vi "are there nodes with unexplored children.vi"(8 "error in (no error)":errorcluster, 11 "current_path":T1[](array[typedef])) -> (0 "error out":errorcluster, 3 "T = there is at least one node with at least one unexplored child":bool)   [LabVIEW 2021, in "Project Euler.lvlib"]
uses:
  Project Euler.lvlib
  lattice_path_node.ctl
  lattice_path_direction.ctl
panel:
  out "node number":i32
  # "Development\ncontrols/indicators useful for development and testing, but which are not outputs of the VI"
  # "Input\nInputs to the VI"
  # "Output\nOutputs of the VI"
  # "Description\n\nBlank VI with error handling case. \n\nSummarize the use of this VI in this space."
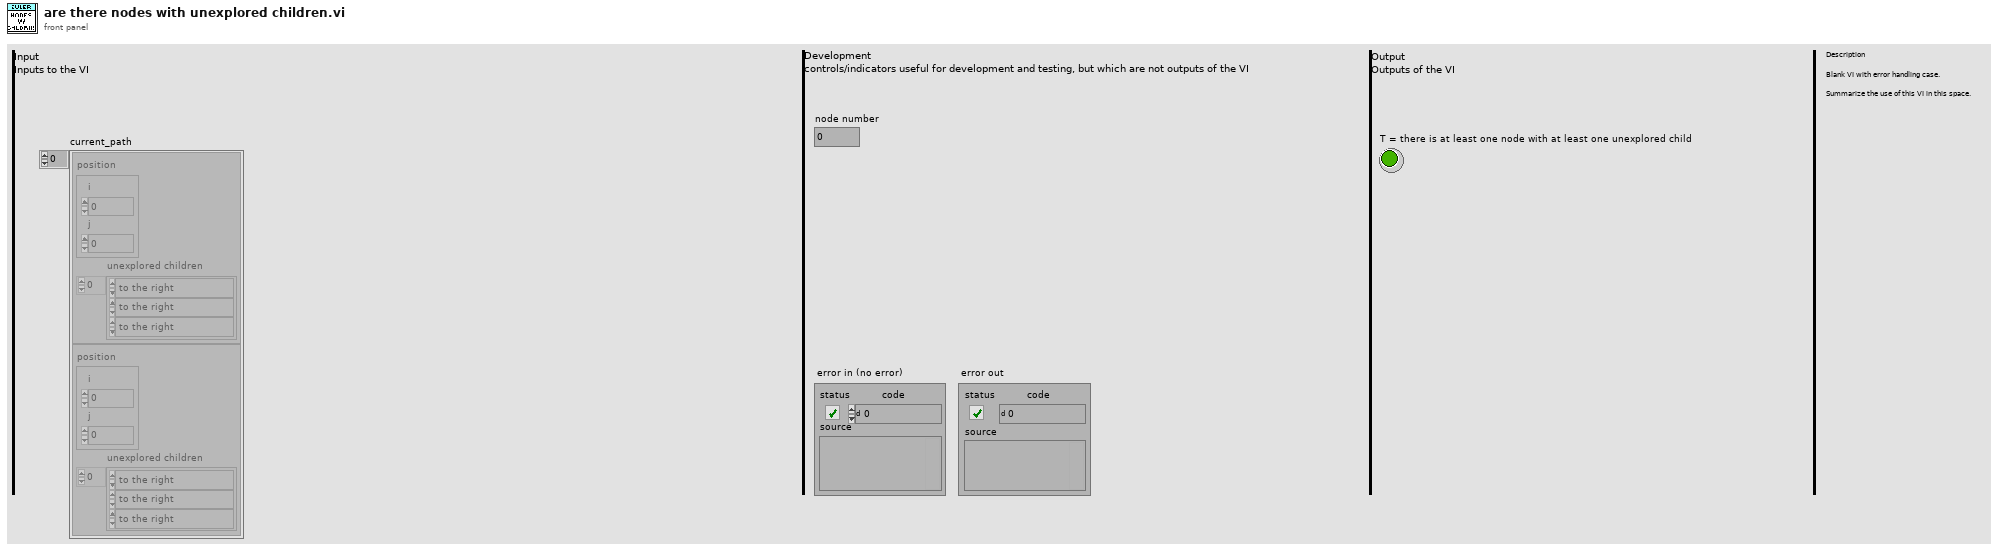
[diagram p1: front panel]
types:
  T1 = typedef "Project Euler.lvlib/lattice_path_node.ctl" = cluster{"position":cluster{"i":i32, "j":i32}, "unexplored children":T2[]}
  T2 = typedef "Project Euler.lvlib/lattice_path_direction.ctl" = enum16{"to the right", "downwards"}
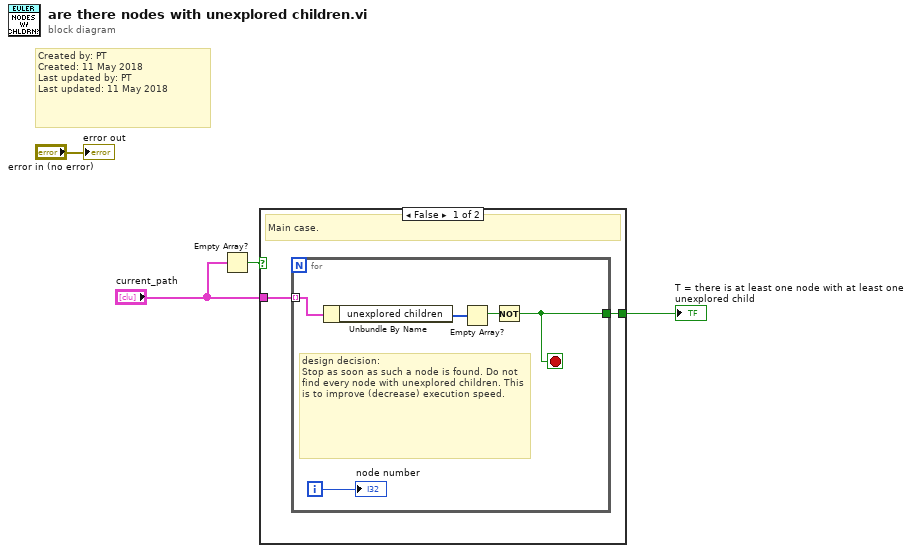
[diagram p0: block diagram]
diagram:
  # "Created by: PT\nCreated: 11 May 2018\nLast updated by: PT\nLast updated: 11 May 2018"
  n1 = Empty Array?(array="current_path") -> (empty?=w2:bool)
  n2 = case shown="False" w2 {
    tunnel: [w6 _] -> w3
    tunnel: "current_path" -> [w5 _]
    frame False {
      # "Main case."
      n3 = for {
        tunnel: w5 -> [w11] mode=indexing
        tunnel: [w8] -> w6
        i -> [w7]
        stop <- w8 stop-if-true
        # "design decision:\nStop as soon as such a node is found. Do not find every node with unexplored children. This is to improve (decrease) execution speed."
        n4 = Unbundle By Name(w11) -> ("unexplored children"=w10:T2[])
        n5 = Empty Array?(array=w10) -> (empty?=w9:bool)
        n6 = Not(x=w9) -> (.not. x?=w8:bool)
        "node number" <- w7
      }
    }
    frame True {
      # "Empty current path"
    }
  }
  "T = there is at least one node with at least one unexplored child" <- w3
  "error out" <- "error in (no error)"
